vi "FGV_MacroGen.vi"(6 "Final Index":i32, 7 "MacroFGV_Commands":T4, 8 "Error In":errorcluster, 9 "Length":i32, 10 "Start Index":i32, 11 "Macro Command IN":T1) -> (0 "Error Out":errorcluster, 2 "Error?":bool, 3 "Macro Cluster Array":T1[](array[typedef]))   [LabVIEW 2012]
doc: "This is the main FGV which manages the Macro Data"
uses:
  FGV_MacroGen_Commands.ctl
  Custom Controls and Typedefs/Macro_CommandStruct.ctl
  Custom Controls and Typedefs/Macro_Action_List.ctl
  Custom Controls and Typedefs/Macro_ArgumentStruct.ctl
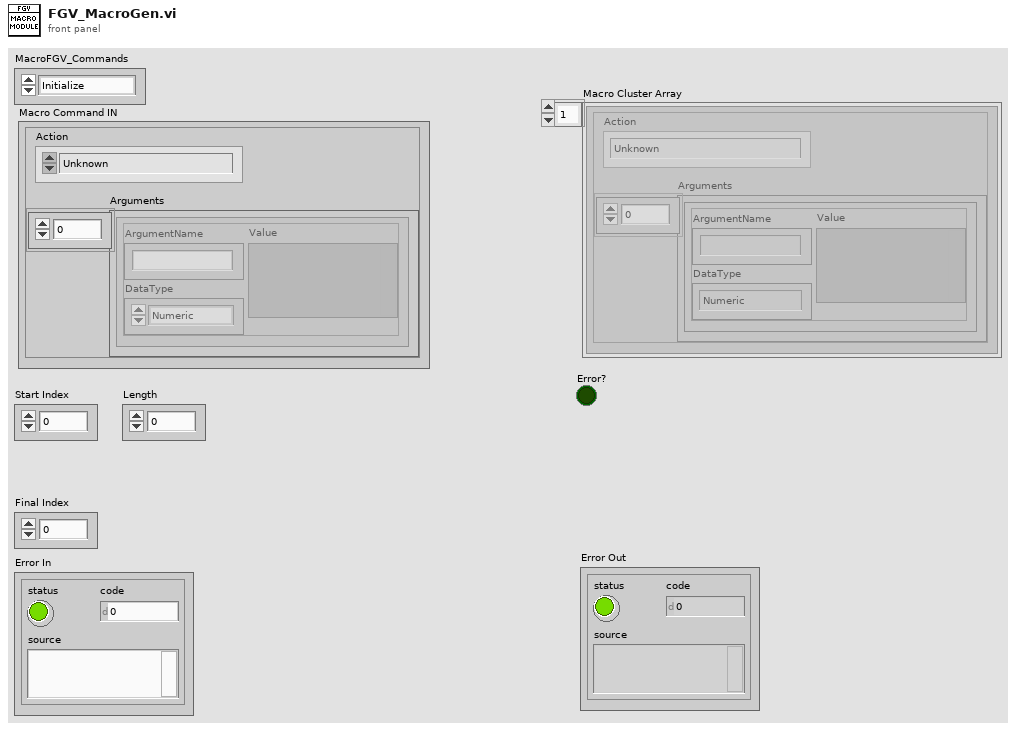
[diagram p1: front panel]
types:
  T1 = typedef "Macro_CommandStruct.ctl" = cluster{"Action":T2, "Arguments":T3[]}
  T2 = typedef "Macro_Action_List.ctl" = enum16{"Unknown", "2D.Frame.Scan", "2D.Line.Scan", "Load.Settings.File", "Move.To.Position", "Pause", "Z.Stack", "LOOP.Start", "LOOP.End"}
  T3 = typedef "Macro_ArgumentStruct.ctl" = cluster{"ArgumentName":string, "DataType":enum16{"Numeric", "String"}, "Value":variant}
  T4 = typedef "FGV_MacroGen_Commands.ctl" = enum16{"Initialize", "Get Array", "Load from file", "Insert Item", "Insert at End", "Edit Item", "Delete Item", "Move Items", "Save", "SaveAs"}
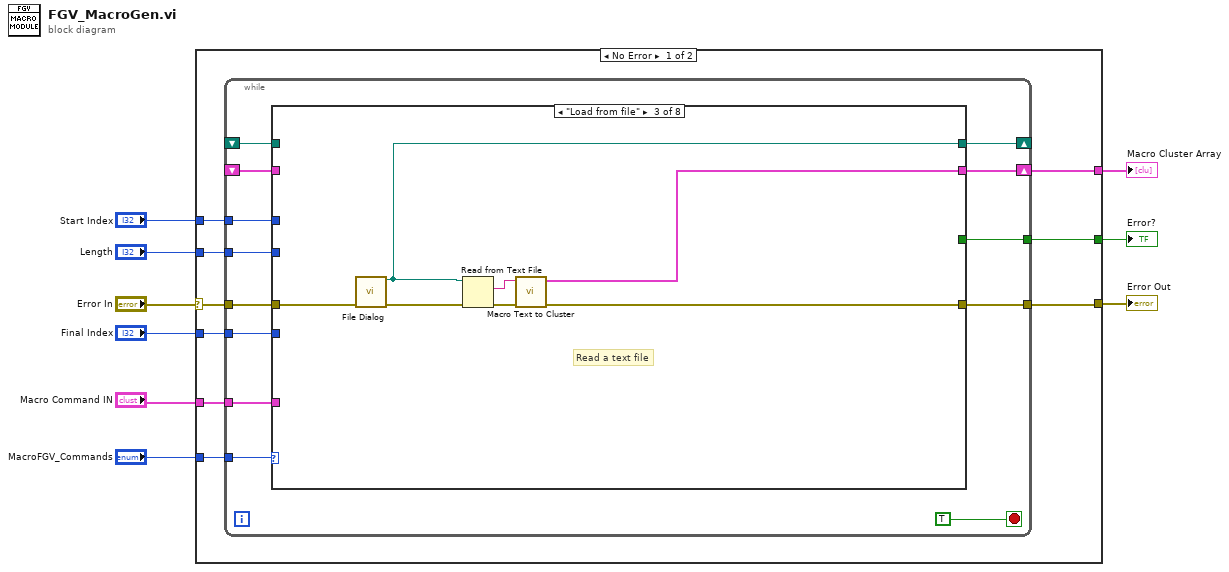
[diagram p0: block diagram]
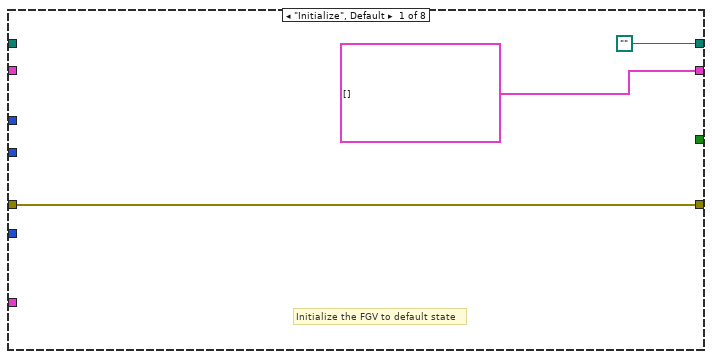
[diagram p2: hidden frame]
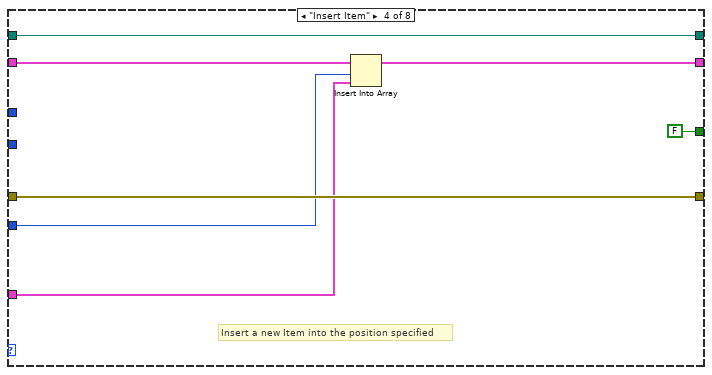
[diagram p4: hidden frame]
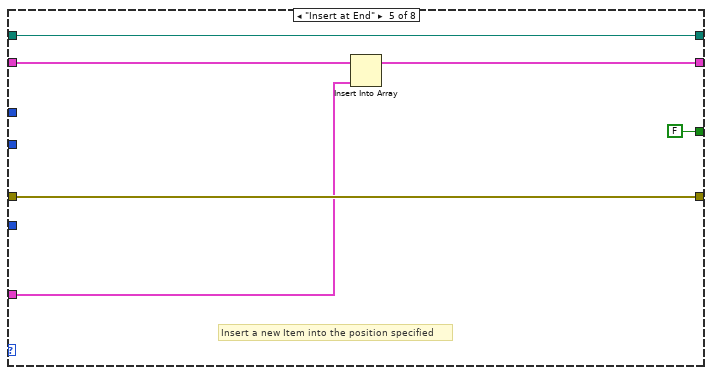
[diagram p5: hidden frame]
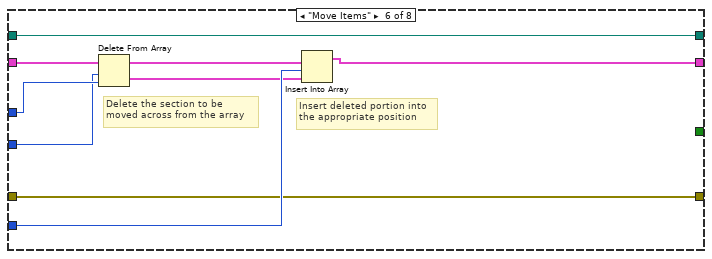
[diagram p6: hidden frame]
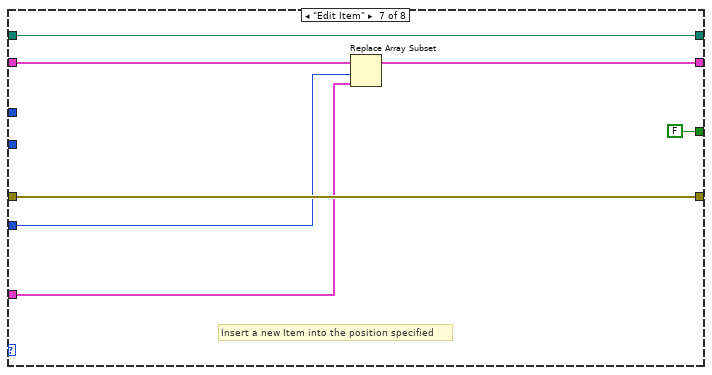
[diagram p7: hidden frame]
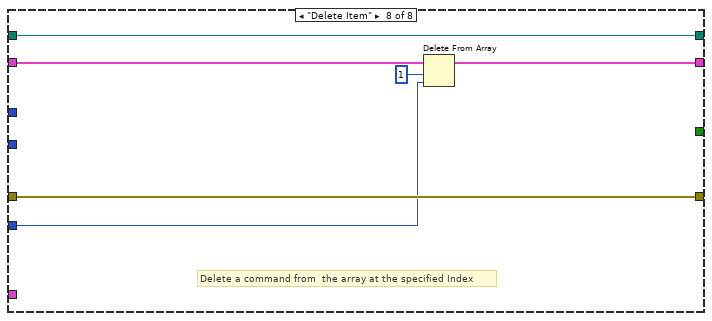
[diagram p8: hidden frame]
diagram:
  n1 = case shown="No Error" "Error In" {
    selector: "Error In" -> [w17 w80]
    tunnel: "MacroFGV_Commands" -> [w18 _]
    tunnel: "Final Index" -> [w16 _]
    tunnel: [w15 _] -> w6
    tunnel: "Macro Command IN" -> [w14 _]
    tunnel: [w13 _] -> w5
    tunnel: [w12 w80] -> w4
    tunnel: "Start Index" -> [w11 _]
    tunnel: "Length" -> [w10 _]
    frame No Error {
      n2 = while {
        tunnel: w18 -> [w30]
        shift-right: [w29] -> _
        shift-left: _ -> [w28]
        tunnel: w17 -> [w27]
        tunnel: w16 -> [w26]
        shift-right: [w25] -> w13
        shift-left: _ -> [w24]
        tunnel: [w23] -> w15
        tunnel: w14 -> [w22]
        tunnel: [w21] -> w12
        tunnel: w11 -> [w20]
        tunnel: w10 -> [w19]
        stop <- TRUE stop-if-true
        n3 = case shown="\"Load from file\"" w30 {
          tunnel: [path "" w37 w38 w51 w57 w66 w73 w79] -> w29
          tunnel: w28 -> [_ w37 _ w51 w57 w66 w73 w79]
          tunnel: w27 -> [w32 w35 w40 w49 w55 w59 w70 w75]
          tunnel: w26 -> [_ _ _ w47 _ w61 w68 w74]
          tunnel: [T1[] [] w36 w41 w50 w56 w58 w71 w76] -> w25
          tunnel: w24 -> [_ w36 _ w45 w52 w65 w72 w78]
          tunnel: [_ _ _ FALSE FALSE _ FALSE _] -> w23
          tunnel: w22 -> [_ _ _ w48 w54 _ w69 _]
          tunnel: [w32 w35 w42 w49 w55 w59 w70 w75] -> w21
          tunnel: w20 -> [_ _ _ _ _ w64 _ _]
          tunnel: w19 -> [_ _ _ _ _ w63 _ _]
          frame "Initialize", Default {
            # "Initialize the FGV to default state"
          }
          frame "Get Array" {
            # "Returns an array of all the stored commands"
          }
          frame "Load from file" {
            # "Read a text file"
            n4 = call "File Dialog"("error in"=w40) -> ("selected path"=w38:path, "error out"=w39:errorcluster)  [unwired: 11 in, 2 out]
            n5 = Read from Text File(file (use dialog)=w38, error in=w39) -> (text=w44:string, error out=w43:errorcluster)  [unwired: 2 in, 2 out]
            n6 = call "Macro Text to Cluster.vi"("Error In"=w43, "Macro Text IN"=w44) -> ("Error Out"=w42:errorcluster, "Macro Cluster Array OUT"=w41:T1[])  [unwired: 8 in]
          }
          frame "Insert Item" {
            # "Insert a new Item into the position specified"
            n7 = Insert Into Array(array=w45, index=w47, new element=w48) -> (w50:T1[])
          }
          frame "Insert at End" {
            # "Insert a new Item into the position specified"
            n8 = Insert Into Array(array=w52, new element=w54) -> (w56:T1[])  [unwired: 1 in]
          }
          frame "Move Items" {
            # "Insert deleted portion into\nthe appropriate position"
            # "Delete the section to be\nmoved across from the array"
            n9 = Delete From Array(array=w65, length=w63, index=w64) -> (deleted portion=w60:T1[], array with subset deleted=w62:T1[])
            n10 = Insert Into Array(array=w62, index=w61, new element=w60) -> (w58:T1[])
          }
          frame "Edit Item" {
            # "Insert a new Item into the position specified"
            n11 = Replace Array Subset(array=w72, new element=w69, index=w68) -> (w71:T1[])
          }
          frame "Delete Item" {
            # "Delete a command from  the array at the specified Index"
            n12 = Delete From Array(array=w78, length=1, index=w74) -> (array with subset deleted=w76:T1[])  [unwired: 1 out]
          }
        }
      }
    }
    frame Error {
    }
  }
  "Error Out" <- w4
  "Error?" <- w6
  "Macro Cluster Array" <- w5
